vi "InitTileFromFile.vi"() -> (0 "Init Data Out":fxp<+,3,3>[](array[numeric]))   [LabVIEW 2019, in "Initializers.lvlib"]
uses:
  Initializers.lvlib
panel:
  out "new picture 2":picture
  in  "path to PNG file":path=path "C:/Users/FreshBob/Dropbox/VIs/myRIO_GameConsole/Data/Tilesets/UnifiedTileset.png"
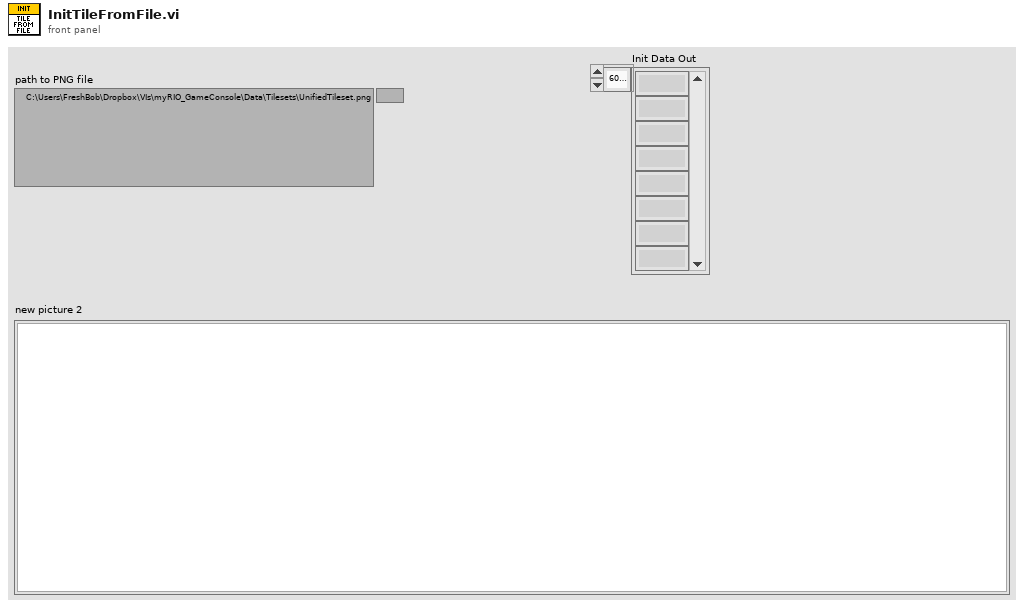
[diagram p1: front panel]
types:
  T1 = typedef "imagedata.ctl" = cluster{"image type":i32, "image depth":i32, "image":u8[], "mask":u8[], "colors":u32[], "Rectangle":cluster{"left":i16, "top":i16, "right":i16, "bottom":i16}}
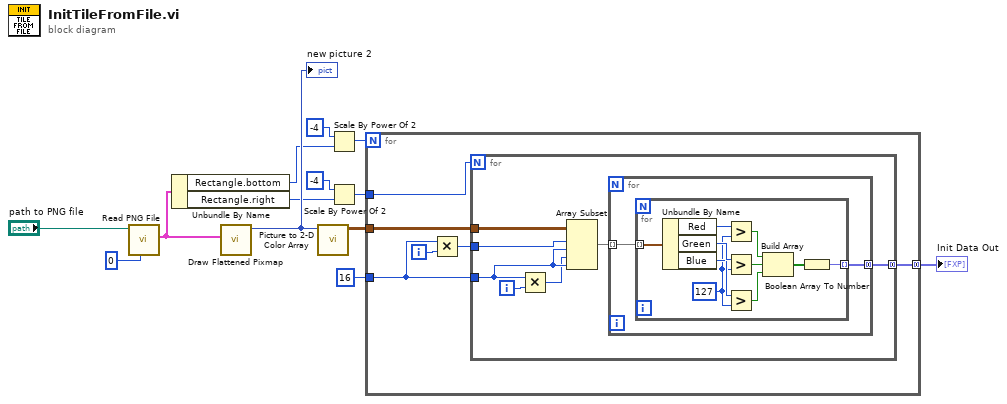
[diagram p0: block diagram]
diagram:
  n1 = call <vilib>:"Read PNG File.vi"("Transparency Thresh"=u8 0, "path to PNG file"="path to PNG file") -> ("image data"=w8:T1)  [unwired: 7 in, 2 out]
  n2 = Unbundle By Name(w8) -> ("Rectangle.bottom"=w7:i16, "Rectangle.right"=w4:i16)
  n3 = call <vilib>:"Draw Flattened Pixmap.vi"("image data"=w8) -> ("new picture"=w10:picture)  [unwired: 8 in]
  "new picture 2" <- w10
  n4 = call "Picture to 2-D Color Array.vi"("picture"=w10) -> ("Color Array"=w13:cluster{"Red":u8, "Green":u8, "Blue":u8}[][])  [unwired: 9 in, 1 out]
  n5 = Scale By Power Of 2(n=i16 -4, x=w7) -> (x*2^n=w2:i16)
  n6 = Scale By Power Of 2(n=i16 -4, x=w4) -> (x*2^n=w3:i16)
  n7 = for {
    N: w2 -> [_]
    tunnel: w13 -> [w19]
    tunnel: 16 ("length") -> [w16]
    tunnel: [w18] -> w1 mode=concatenating
    tunnel: w3 -> [w14]
    i -> [w17]
    n8 = Multiply(x=w16, y=w17) -> (x*y=w15:i32)
    n9 = for {
      N: w14 -> [_]
      tunnel: w19 -> [w26]
      tunnel: w16 -> [w24]
      tunnel: [w23] -> w18 mode=concatenating
      tunnel: w15 -> [w20]
      i -> [w25]
      n10 = Multiply(x=w24, y=w25) -> (x*y=w21:i32)
      n11 = Array Subset(array=w26, index (row)=w20, length (row)=w24, index (col)=w21, length (col)=w24) -> (w22:cluster{"Red":u8, "Green":u8, "Blue":u8}[][])
      n12 = for {
        tunnel: w22 -> [w28] mode=indexing
        tunnel: [w27] -> w23 mode=concatenating
        n13 = for {
          tunnel: w28 -> [w38] mode=indexing
          tunnel: [w32] -> w27 mode=indexing
          w34 = u8 127 ("y")
          n14 = Unbundle By Name(w38) -> ("Red"=w37:u8, "Green"=w36:u8, "Blue"=w35:u8)
          n15 = Greater?(x=w37, y=w34) -> (0:w31:bool)
          n16 = Greater?(x=w36, y=w34) -> (0:w30:bool)
          n17 = Greater?(x=w35, y=w34) -> (0:w29:bool)
          n18 = Build Array(w31, w30, w29) -> (w33:bool[])
          n19 = Boolean Array To Number(Boolean array=w33) -> (number=w32:fxp<+,3,3>)
        }
      }
    }
  }
  "Init Data Out" <- w1
